vi "_readtemp.vi"(8 "error in (no error)":errorcluster) -> (0 "error out":errorcluster, 2 "Temperature":dbl)   [LabVIEW 2018]
doc: "VI simuleerib temperatuuri mõõtmist. Veaklastrid on ainult andmevoo juhtimiseks ja ei mõjuta VI tööd."
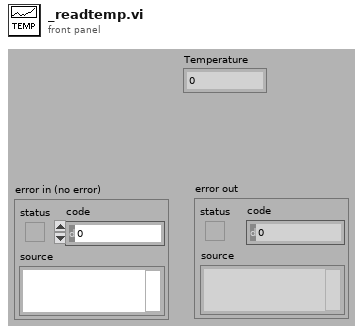
[diagram p1: front panel]
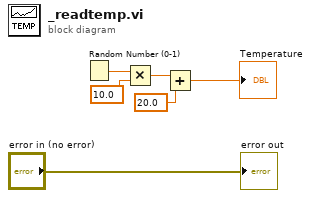
[diagram p0: block diagram]
diagram:
  n1 = Random Number (0-1)() -> (number: 0 to 1=w6:dbl)
  n2 = Multiply(x=w6, y=10.0) -> (x*y=w4:dbl)
  n3 = Add(x=w4, y=20.0) -> (x+y=→"Temperature":dbl)
  "error out" <- "error in (no error)"
